vi "Get SysCfg Device Information.vi"(8 "error in":errorcluster, 11 "SysCfg Device in":refnum<class "SysCfg Device.lvclass">) -> (0 "error out":errorcluster, 2 "Device Information":T1 {"Product ID" format="%.0x"}, 3 "SysCfg Device out":refnum<class "SysCfg Device.lvclass">)   [LabVIEW 2015, in "SMI.lvlib" / "SysCfg Device.lvclass"]
uses:
  SysCfg Device.lvclass
  Controls/SysCfgDeviceInformation.ctl
  SysCfg Device.lvclass/SysCfg Device.ctl
  Device/Device.lvclass/Device.ctl
  Accessor Methods/Read SysCfg Session.vi
  Device/Accessor Methods/Read Vendor Name.vi
  Device/Accessor Methods/Read Product Name.vi
  Device/Accessor Methods/Read Product ID.vi
  Device/Accessor Methods/Read Serial Number.vi
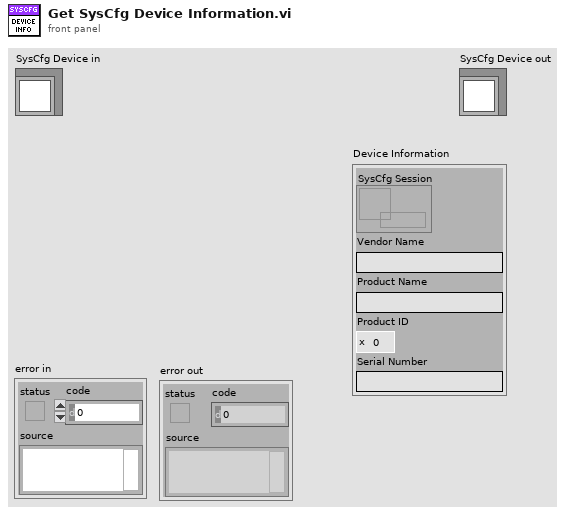
[diagram p1: front panel]
types:
  T1 = typedef "SMI.lvlib/SysCfg Device.lvclass/SysCfgDeviceInformation.ctl" = cluster{"SysCfg Session":refnum<data-value>, "Vendor Name":string, "Product Name":string, "Product ID":u32, "Serial Number":string}
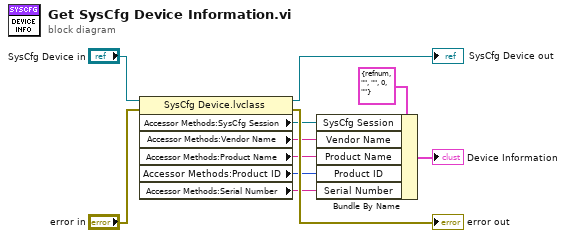
[diagram p0: block diagram]
diagram:
  n1 = property class="SysCfg Device.lvclass"(reference="SysCfg Device in", error in="error in") -> (reference out=→"SysCfg Device out":refnum<class "SysCfg Device.lvclass">, error out=→"error out":errorcluster, "Accessor Methods:SysCfg Session"=w5:refnum<data-value>, "Accessor Methods:Vendor Name"=w4:string, "Accessor Methods:Product Name"=w3:string, "Accessor Methods:Product ID"=w2:u16, "Accessor Methods:Serial Number"=w1:string)
  n2 = Bundle By Name(cluster=T1 {"SysCfg Session"=refnum, "Vendor Name"="", "Product Name"="", "Product ID"=0, "Serial Number"=""} ("Device Information"), "SysCfg Session"=w5, "Vendor Name"=w4, "Product Name"=w3, "Product ID"=w2, "Serial Number"=w1) -> (→"Device Information":T1)
